vi "PseudoHeart.vi"() -> ()   [LabVIEW 2020]
uses:
  <vilib>/Analysis/NI_AAL_SigProc.lvlib
panel:
  out "?":dynamicdata(graph)
  out "Waveform Chart":dynamicdata(graph)
  in  "stop":bool
  out "Heart Monitering":dbl
  out "Frequency in hertz":dbl
  out "Scalar":dbl
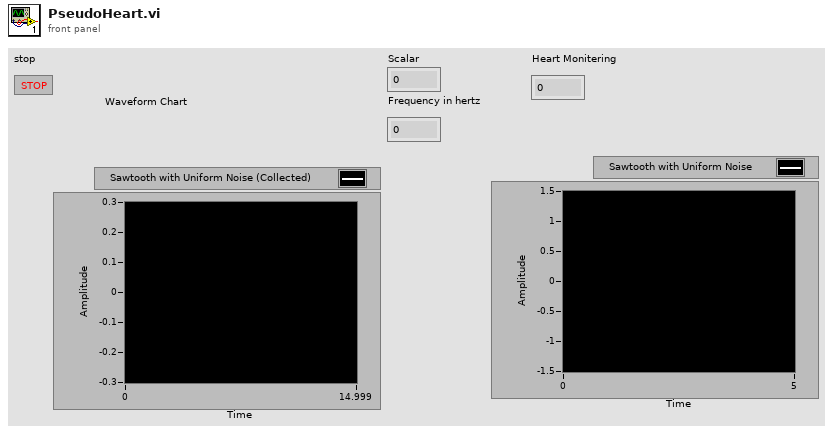
[diagram p1: front panel]
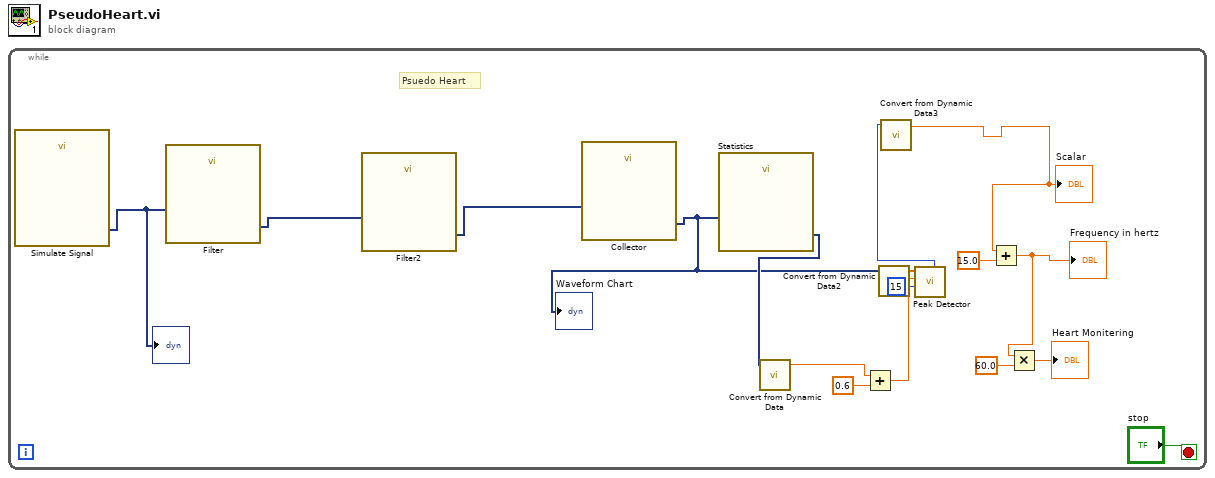
[diagram p0: block diagram]
diagram:
  n1 = while {
    stop <- "stop" stop-if-true
    # "Psuedo Heart"
    n2 = call "Simulate Signal"() -> ("Sawtooth with Uniform Noise"=w4:dynamicdata)  [unwired: 14 in, 1 out]
    "?" <- w4
    n3 = call "Filter"("Signal"=w4) -> ("Filtered Signal"=w17:dynamicdata)  [unwired: 9 in, 1 out]
    n4 = call "Filter2"("Signal"=w17) -> ("Filtered Signal"=w16:dynamicdata)  [unwired: 9 in, 1 out]
    n5 = call "Collector"("Signals"=w16) -> ("Collected Signals"=w1:dynamicdata)  [unwired: 9 in, 1 out]
    "Waveform Chart" <- w1
    n6 = call "Statistics"("Signals"=w1) -> ("Maximum"=w3:dynamicdata)  [unwired: 25 in, 1 out]
    n7 = call "Convert from Dynamic Data"("Dynamic Data Type"=w3) -> ("Scalar"=w14:dbl)  [unwired: 3 in]
    n8 = Add(x=w14, y=0.6) -> (x+y=w13:dbl)
    n9 = call "Convert from Dynamic Data2"("Dynamic Data Type"=w1) -> ("Array"=w2:dbl[])  [unwired: 3 in]
    n10 = call <vilib>:"Peak Detector.vi"("width"=15, "threshold"=w13, "X"=w2) -> ("# found"=w7:i32)  [unwired: 4 in, 4 out]
    n11 = call "Convert from Dynamic Data3"("Dynamic Data Type"=w7) -> ("Scalar"=w6:dbl)  [unwired: 3 in]
    "Scalar" <- w6
    n12 = Add(x=w6, y=15.0) -> (x+y=w10:dbl)
    "Frequency in hertz" <- w10
    n13 = Multiply(x=w10, y=60.0) -> (x*y=→"Heart Monitering":dbl)
  }
